vi "Setup UI.vi"(8 "error in (no error)":errorcluster, 10 "Set UI to input? (F)":bool, 11 "PC Reader.lvclass":refnum<class "Photon Counter Reader.lvclass">) -> (0 "error out":errorcluster, 3 "PC Reader out":refnum<class "Photon Counter Reader.lvclass">)   [LabVIEW 2017, in "Photon Counter Reader.lvclass"]
doc: "Setup UI (re)constructs an object -- populates its member data -- from a front panel the user can see. The VI should be as simple as possible so that a UI loop can poll it continuously for updates. \n\nThe VI is designed to be used as a subPanel within another VI. Wire true to \"Set UI to input\" only on the first call, just after inserting this VI into a subPanel, to populate its controls with the class's current values.\n\nSetup UI is distinct from the class constructor. Class constructors are not polymorphic, yet configure dialogs need to configure objects without knowing their type -- and polymorphism is the necessary solution. Thus, Setup UI is a polymorphic class constructor. This continously polled \"Setup UI\" concept is a kludge: a better idea would be an XControl, but those require a steeper learning curve."
uses:
  Photon Counter Reader.lvclass
  Photon Counter Reader.lvclass/Photon Counter Reader.ctl
panel:
  in  "clear template":bool
  in  "Which channels?":u16(ring)=2 items=["A", "B", "A and B", "A, B average"]
  in  "template: Ch A scan":bool
  in  "template: Ch A/B split":bool
  in  "template: continuous scan":bool
  in  "Gate B Ref":enum16{"t=0", "t=T/4", "t=T/2", "t=3T/4"}(ring)
  in  "Gate A Ref":enum16{"t=0", "t=T/4", "t=T/2", "t=3T/4"}(ring)
  out "Gate B Delay Actual":dbl[unit]
  out "Gate A Delay Actual":dbl[unit]
  in  "start vs mid. of gate":bool caption="Delays measured to"
  in  "Gate B %":dbl
  in  "Gate A %":dbl
  in  "time vs percent":bool caption="Width in"
  out "Gate B Mode":enum16{"CW", "Fixed", "Scan"}(ring)
  out "Gate A Mode":enum16{"CW", "Fixed", "Scan"}(ring)
  in  "Gate B Width":dbl[unit]
  in  "Gate B Delay":dbl[unit]
  in  "Gate A Delay":dbl[unit]
  in  "Gate A Width":dbl[unit]
  in  "Ext. Trigger?":bool
  in  "Ext. Trig. Freq.":dbl[unit]=42076.2
  in  "Count Time":dbl[unit]=1.0 format="%#_4g"
  in  "Send first pt to PC":bool
  in  "indAw?":bool
  in  "indAd?":bool
  in  "indBw?":bool
  in  "indBd?":bool
  # "Photon Counter Setup"
  # "Track ind.var.?\n(assumes in ns)"
  # "(PEM = 42.0762 kHz)"
  # "(If tracking, these times represent \nthe values for the first pt.)"
  # "PURE VIRTUAL\nMETHOD CALLED!"
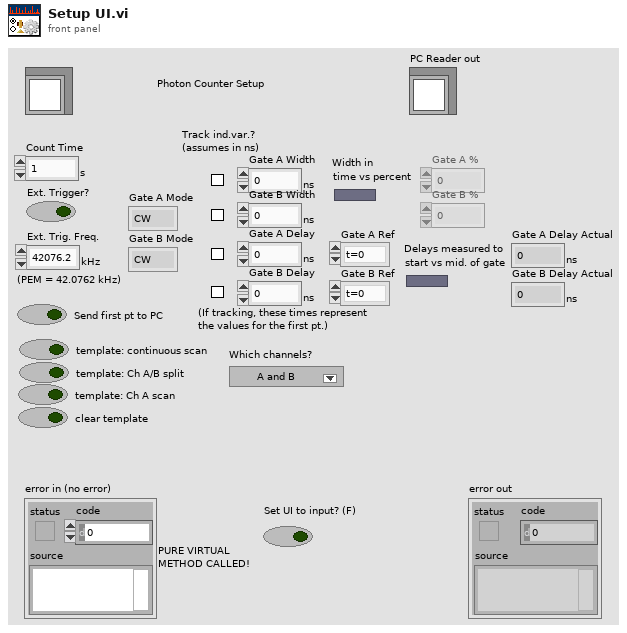
[diagram p1: front panel]
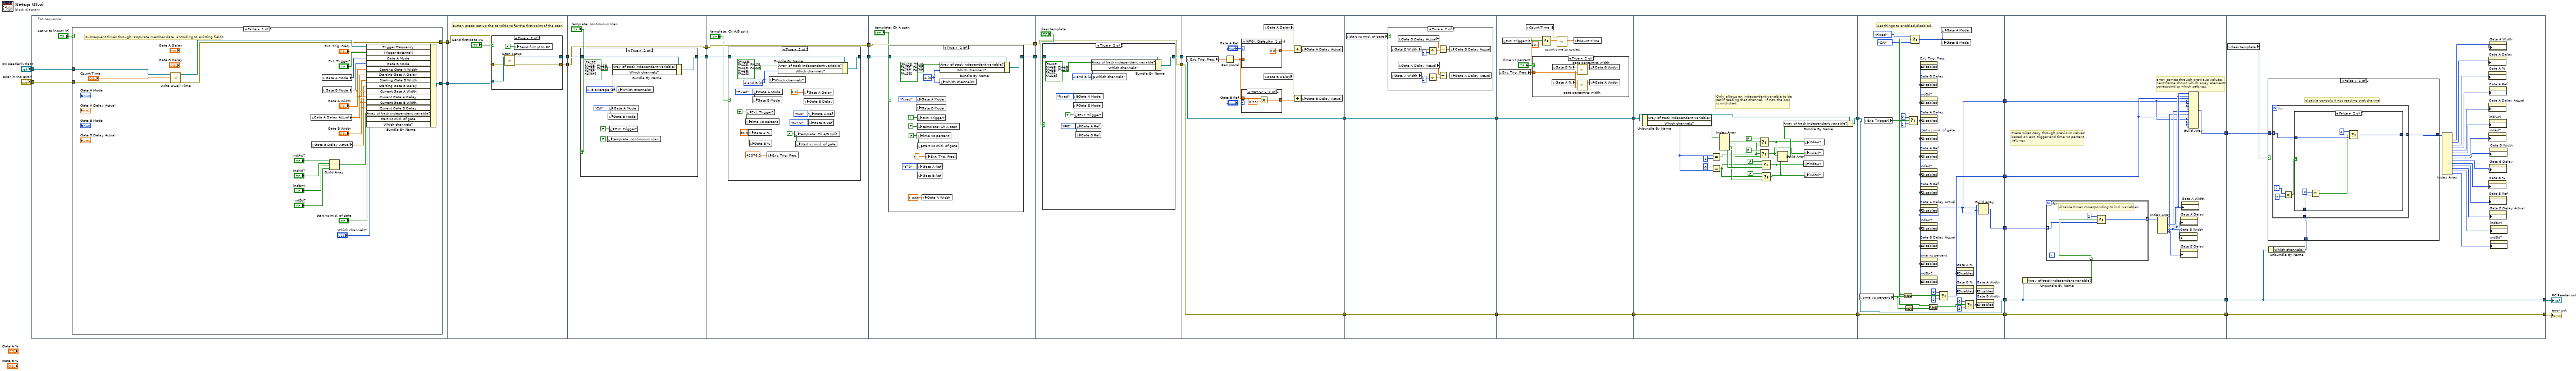
[diagram p0: block diagram]
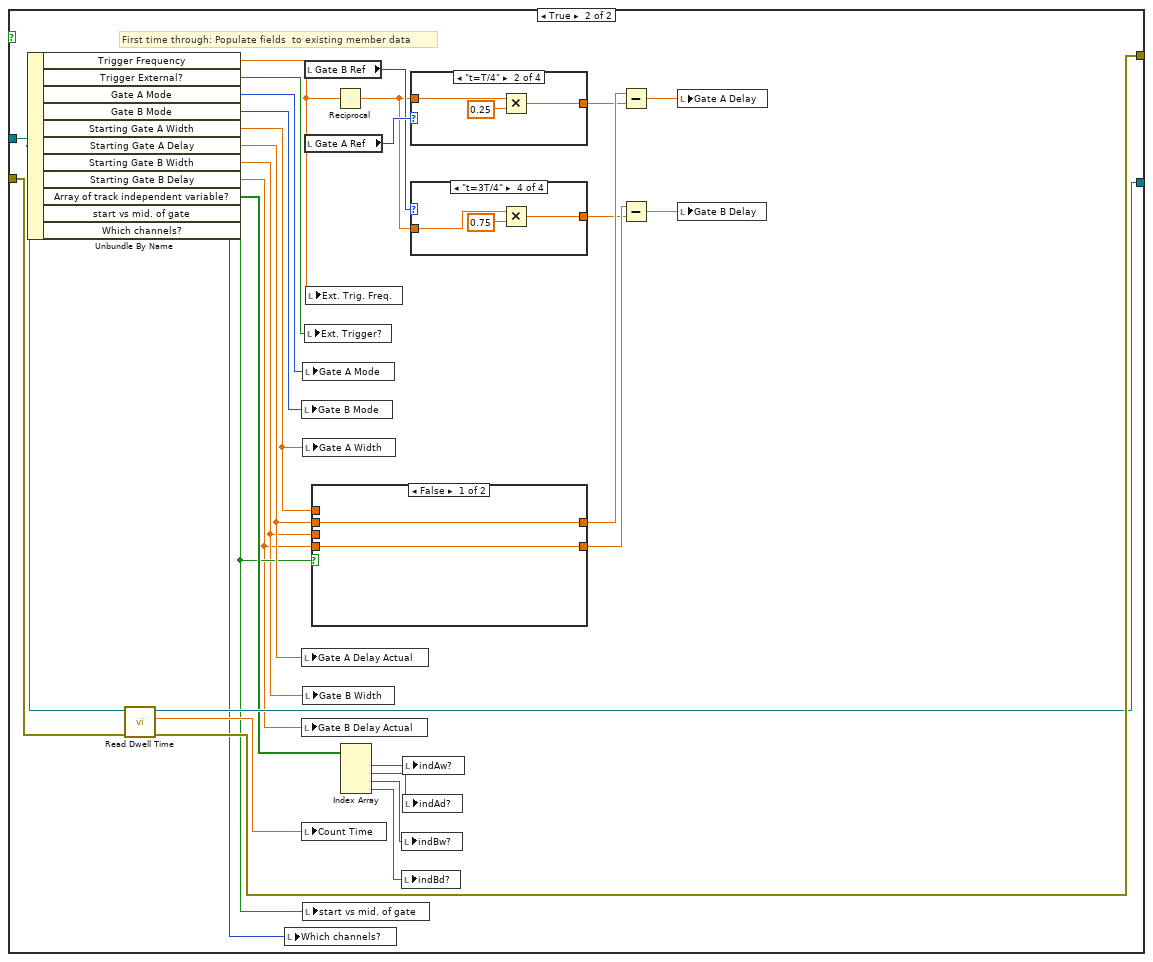
[diagram p2: hidden frame]
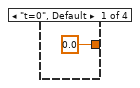
[diagram p3: hidden frame]
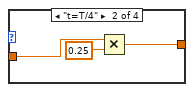
[diagram p4: hidden frame]
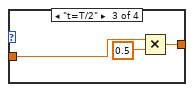
[diagram p5: hidden frame]
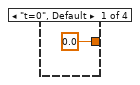
[diagram p6: hidden frame]
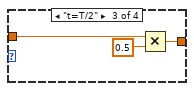
[diagram p7: hidden frame]
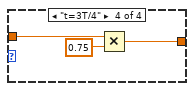
[diagram p8: hidden frame]
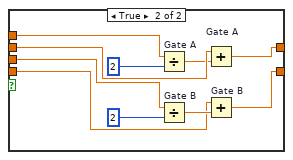
[diagram p9: hidden frame]
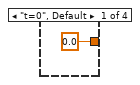
[diagram p15: hidden frame]
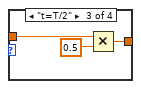
[diagram p16: hidden frame]
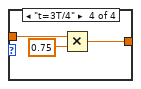
[diagram p17: hidden frame]
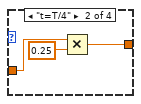
[diagram p18: hidden frame]
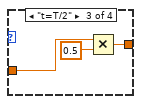
[diagram p19: hidden frame]
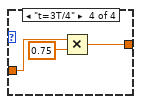
[diagram p20: hidden frame]
diagram:
  n1 = flat-sequence {
    tunnel: "error in (no error)" -> [w34]
    tunnel: [w37] -> w26
    tunnel: [w33] -> w25
    tunnel: "PC Reader.lvclass" -> [w35]
    tunnel: w26 -> [w124]
    tunnel: w25 -> [w123]
    tunnel: [w122] -> w24
    tunnel: [w120] -> w23
    tunnel: w24 -> [w132]
    tunnel: w23 -> [w134]
    tunnel: [w133] -> w22
    tunnel: [w132] -> w21
    tunnel: w22 -> [w145]
    tunnel: [w144] -> w20
    tunnel: w21 -> [w146]
    tunnel: [w146] -> w19
    tunnel: w20 -> [w163]
    tunnel: [w162] -> w4
    tunnel: w19 -> [w164]
    tunnel: [w164] -> w2
    tunnel: w4 -> [w178]
    tunnel: [w179] -> w3
    tunnel: w2 -> [w177]
    tunnel: [w177] -> w1
    tunnel: [w200] -> w29
    tunnel: [w199] -> w28
    tunnel: w3 -> [w199]
    tunnel: w1 -> [w200]
    tunnel: w29 -> [w223]
    tunnel: [w223] -> w31
    tunnel: w28 -> [w222]
    tunnel: [w222] -> w30
    tunnel: w31 -> [w244]
    tunnel: [w244] -> w18
    tunnel: w30 -> [w243]
    tunnel: [w243] -> w16
    tunnel: w18 -> [w276]
    tunnel: [w276] -> w17
    tunnel: w16 -> [w261]
    tunnel: [w260] -> w15
    tunnel: w17 -> [w286]
    tunnel: w15 -> [w285]
    tunnel: [w286] -> w12
    tunnel: [w285] -> w11
    tunnel: [w284] -> w10
    tunnel: [w282] -> w9
    tunnel: [w281] -> w8
    tunnel: w12 -> [w308]
    tunnel: w11 -> [w306]
    tunnel: w10 -> [w304]
    tunnel: w9 -> [w299]
    tunnel: w8 -> [w298]
    tunnel: [w308] -> w7
    tunnel: [w306] -> w6
    tunnel: [w297] -> w5
    tunnel: [w331] -> w13
    tunnel: [w332] -> w14
    tunnel: w7 -> [w332]
    tunnel: w6 -> [w331]
    tunnel: w5 -> [w329]
    frame #0 {
      n2 = case shown="False" "Set UI to input? (F)" {
        tunnel: [w50 w78] -> w37
        tunnel: w35 -> [w51 w79]
        tunnel: [w47 w80] -> w33
        tunnel: w34 -> [w46 w81]
        frame False {
          # "Subsequent times through: Populate member data  according to existing fields"
          n3 = call-dynamic "Write Dwell Time.vi"("error in (no error)"=w46, "Dwell Time"="Count Time", "Reader.lvclass in"=w51) -> ("error out"=w47:errorcluster, "Reader.lvclass out"=w49:refnum<class "Photon Counter Reader.lvclass">)  [unwired: 7 out]
          n4 = local read "Gate A Delay Actual"() -> (w43:dbl[unit])
          n5 = local read "Gate B Delay Actual"() -> (w41:dbl[unit])
          n6 = local read "Gate A Mode"() -> (w52:enum16{"CW", "Fixed", "Scan"})
          n7 = local read "Gate B Mode"() -> (w45:enum16{"CW", "Fixed", "Scan"})
          n8 = Build Array("indAw?", "indAd?", "indBw?", "indBd?") -> (w40:bool[])
          n9 = Bundle By Name(cluster=w49, "Trigger Frequency"="Ext. Trig. Freq.", "Trigger External?"="Ext. Trigger?", "Gate A Mode"=w52, "Gate B Mode"=w45, "Starting Gate A Width"="Gate A Width", "Starting Gate A Delay"=w43, "Starting Gate B Width"="Gate B Width", "Starting Gate B Delay"=w41, "Current Gate A Width"="Gate A Width", "Current Gate A Delay"=w43, "Current Gate B Width"="Gate B Width", "Current Gate B Delay"=w41, "Array of track independent variable?"=w40, "start vs mid. of gate"="start vs mid. of gate", "Which channels?"="Which channels?") -> (w50:refnum<class "Photon Counter Reader.lvclass">)
        }
        frame True {
          # "First time through: Populate fields  to existing member data"
          n10 = Unbundle By Name(w79) -> ("Trigger Frequency"=w74:dbl[unit], "Trigger External?"=w83:bool, "Gate A Mode"=w82:u16, "Gate B Mode"=w68:u16, "Starting Gate A Width"=w66:dbl[unit], "Starting Gate A Delay"=w67:dbl[unit], "Starting Gate B Width"=w63:dbl[unit], "Starting Gate B Delay"=w62:dbl[unit], "Array of track independent variable?"=w65:bool[], "start vs mid. of gate"=w64:bool, "Which channels?"=w59:u16)
          n11 = call-dynamic "Read Dwell Time.vi"("error in (no error)"=w81, "Reader.lvclass in"=w79) -> ("error out"=w80:errorcluster, "Dwell Time"=w77:dbl[unit], "Reader.lvclass out"=w78:refnum<class "Photon Counter Reader.lvclass">)  [unwired: 7 out]
          n12 = local write "Which channels?"(w59) -> ()
          n13 = local write "Gate B Mode"(w68) -> ()
          n14 = local write "Gate A Delay Actual"(w67) -> ()
          n15 = local write "Gate B Delay Actual"(w62) -> ()
          n16 = local write "Count Time"(w77) -> ()
          n17 = local write "Gate A Mode"(w82) -> ()
          n18 = local write "Gate A Width"(w66) -> ()
          n19 = local write "Gate B Width"(w63) -> ()
          n20 = local write "start vs mid. of gate"(w64) -> ()
          n21 = local read "Gate B Ref"() -> (w75:enum16{"t=0", "t=T/4", "t=T/2", "t=3T/4"})
          n22 = local read "Gate A Ref"() -> (w76:enum16{"t=0", "t=T/4", "t=T/2", "t=3T/4"})
          n23 = local write "Ext. Trigger?"(w83) -> ()
          n24 = local write "Ext. Trig. Freq."(w74) -> ()
          n25 = case shown="False" w64 {
            tunnel: [w109 w113] -> w72
            tunnel: w67 -> [w109 w117]
            tunnel: [w108 w112] -> w69
            tunnel: w66 -> [_ w114]
            tunnel: w63 -> [_ w111]
            tunnel: w62 -> [w108 w110]
            frame False {
            }
            frame True {
              n26 = Divide "Gate A"(x=w114, y=2) -> (x/y=w116:dbl[unit])
              n27 = Divide "Gate B"(x=w111, y=2) -> (x/y=w115:dbl[unit])
              n28 = Add "Gate A"(x=w117, y=w116) -> (x+y=w113:dbl[unit])
              n29 = Add "Gate B"(x=w110, y=w115) -> (x+y=w112:dbl[unit])
            }
          }
          n30 = Reciprocal(x=w74) -> (1/x=w73:dbl[unit])
          n31 = Index Array(array=w65) -> (element #1=w84:bool, element #2=w85:bool, element #3=w86:bool, element #4=w87:bool)  [unwired: 4 in]
          n32 = local write "indBw?"(w86) -> ()
          n33 = local write "indBd?"(w87) -> ()
          n34 = local write "indAw?"(w84) -> ()
          n35 = local write "indAd?"(w85) -> ()
          n36 = case shown="\"t=T/4\"" w76 {
            tunnel: [dbl[unit] 0.0 ("x/y") w99 w102 w105] -> w71
            tunnel: w73 -> [_ w100 w103 w106]
            frame "t=0", Default {
            }
            frame "t=T/4" {
              n37 = Multiply(x=w100, y=0.25) -> (x*y=w99:dbl[unit])
            }
            frame "t=T/2" {
              n38 = Multiply(x=w103, y=0.5) -> (x*y=w102:dbl[unit])
            }
            frame "t=3T/4" {
              n39 = Multiply(x=w106, y=0.75) -> (x*y=w105:dbl[unit])
            }
          }
          n40 = case shown="\"t=3T/4\"" w75 {
            tunnel: [dbl[unit] 0.0 ("x/y") w89 w92 w95] -> w60
            tunnel: w73 -> [_ w90 w93 w96]
            frame "t=0", Default {
            }
            frame "t=T/4" {
              n41 = Multiply(x=w90, y=0.25) -> (x*y=w89:dbl[unit])
            }
            frame "t=T/2" {
              n42 = Multiply(x=w93, y=0.5) -> (x*y=w92:dbl[unit])
            }
            frame "t=3T/4" {
              n43 = Multiply(x=w96, y=0.75) -> (x*y=w95:dbl[unit])
            }
          }
          n44 = Subtract(x=w72, y=w71) -> (x-y=w70:dbl[unit])
          n45 = Subtract(x=w69, y=w60) -> (x-y=w61:dbl[unit])
          n46 = local write "Gate A Delay"(w70) -> ()
          n47 = local write "Gate B Delay"(w61) -> ()
        }
      }
    }
    frame #1 {
      # "Button press: set up the conditions for the first point of the scan"
      n48 = case shown="True" "Send first pt to PC" {
        tunnel: [w126 w127] -> w120
        tunnel: [w125 w128] -> w122
        tunnel: w124 -> [w126 w130]
        tunnel: w123 -> [w125 w129]
        frame False {
        }
        frame True {
          n49 = call-dynamic "Scan Setup.vi"("error in (no error)"=w129, "PC Reader in"=w130) -> ("error out"=w128:errorcluster, "PC Reader out"=w127:refnum<class "Photon Counter Reader.lvclass">)  [unwired: 8 out]
          n50 = local write "Send first pt to PC"(FALSE ("Send conds for first point to PG")) -> ()
        }
      }
    }
    frame #2 {
      n51 = case shown="True" "template: continuous scan" {
        tunnel: w134 -> [w136 w142]
        tunnel: [w136 w140] -> w133
        frame False {
        }
        frame True {
          w137 = u16 3 items=["A", "B", "A and B", "A, B average"] ("Which channels?")
          w143 = enum16{"CW", "Fixed", "Scan"}."CW" ("Gate A Mode")
          n52 = local write "template: continuous scan"(FALSE ("template: continuous scan")) -> ()
          n53 = local write "Gate B Mode"(w143) -> ()
          n54 = local write "Gate A Mode"(w143) -> ()
          n55 = local write "Ext. Trigger?"(FALSE ("Ext. Trigger?")) -> ()
          n56 = Bundle By Name(cluster=w142, "Array of track independent variable?"=bool[] [FALSE, FALSE, FALSE, FALSE, FALSE, FALSE, FALSE], "Which channels?"=w137) -> (w140:refnum<class "Photon Counter Reader.lvclass">)
          n57 = local write "Which channels?"(w137) -> ()
        }
      }
    }
    frame #3 {
      n58 = case shown="True" "template: Ch A/B split" {
        tunnel: w145 -> [w148 w160]
        tunnel: [w148 w159] -> w144
        frame False {
        }
        frame True {
          w149 = u16 2 items=["A", "B", "A and B", "A, B average"] ("Which channels?")
          w151 = FALSE ("template: Ch A/B split")
          w155 = dbl[unit] 0.0 ("Gate A Delay")
          w156 = 50.0 ("Gate A %")
          w157 = TRUE ("Ext. Trigger?")
          w158 = enum16{"CW", "Fixed", "Scan"}."Fixed" ("Gate A Mode")
          n59 = local write "time vs percent"(w157) -> ()
          n60 = local write "Ext. Trigger?"(w157) -> ()
          n61 = local write "Gate A %"(w156) -> ()
          n62 = local write "Gate B %"(w156) -> ()
          n63 = local write "Gate B Mode"(w158) -> ()
          n64 = local write "Gate A Mode"(w158) -> ()
          n65 = local write "Ext. Trig. Freq."(dbl[unit] 42076.2 ("Ext. Trig. Freq.")) -> ()
          n66 = local write "Which channels?"(w149) -> ()
          n67 = Bundle By Name(cluster=w160, "Array of track independent variable?"=bool[] [FALSE, FALSE, FALSE, FALSE, FALSE, FALSE, FALSE], "Which channels?"=w149) -> (w159:refnum<class "Photon Counter Reader.lvclass">)
          n68 = local write "template: Ch A/B split"(w151) -> ()
          n69 = local write "start vs mid. of gate"(w151) -> ()
          n70 = local write "Gate A Delay"(w155) -> ()
          n71 = local write "Gate B Delay"(w155) -> ()
          n72 = local write "Gate B Ref"(enum16{"t=0", "t=T/4", "t=T/2", "t=3T/4"}."t=T/2" ("Gate B Ref")) -> ()
          n73 = local write "Gate A Ref"(enum16{"t=0", "t=T/4", "t=T/2", "t=3T/4"}."t=0" ("Gate A Ref")) -> ()
        }
      }
    }
    frame #4 {
      n74 = case shown="True" "template: Ch A scan" {
        tunnel: w163 -> [w165 w176]
        tunnel: [w165 w175] -> w162
        frame False {
        }
        frame True {
          w166 = u16 0 items=["A", "B", "A and B", "A, B average"] ("Which channels?")
          w170 = enum16{"t=0", "t=T/4", "t=T/2", "t=3T/4"}."t=0" ("Gate A Ref")
          w169 = FALSE ("time vs percent")
          w174 = enum16{"CW", "Fixed", "Scan"}."Fixed" ("Gate A Mode")
          n75 = local write "Gate A Mode"(w174) -> ()
          n76 = local write "Gate B Mode"(w174) -> ()
          n77 = local write "time vs percent"(w169) -> ()
          n78 = local write "Ext. Trigger?"(TRUE ("Ext. Trigger?")) -> ()
          n79 = local write "template: Ch A scan"(FALSE ("template: Ch A sweep")) -> ()
          n80 = local write "Gate A Ref"(w170) -> ()
          n81 = local write "Gate B Ref"(w170) -> ()
          n82 = local write "start vs mid. of gate"(w169) -> ()
          n83 = local write "Gate A Width"(dbl[unit] 1.0000000000000002e-06 ("Gate A Width")) -> ()
          n84 = local write "Ext. Trig. Freq."(dbl[unit] 1000.0 ("Ext. Trig. Freq.")) -> ()
          n85 = local write "Which channels?"(w166) -> ()
          n86 = Bundle By Name(cluster=w176, "Array of track independent variable?"=bool[] [FALSE, TRUE, FALSE, FALSE, FALSE, FALSE, FALSE], "Which channels?"=w166) -> (w175:refnum<class "Photon Counter Reader.lvclass">)
        }
      }
    }
    frame #5 {
      n87 = case shown="True" "clear template" {
        tunnel: [w181 w187] -> w179
        tunnel: w178 -> [w181 w188]
        frame False {
        }
        frame True {
          w182 = enum16{"t=0", "t=T/4", "t=T/2", "t=3T/4"}."t=0" ("Gate A Ref")
          w183 = enum16{"CW", "Fixed", "Scan"}."Fixed" ("Gate A Mode")
          w185 = u16 2 items=["A", "B", "A and B", "A, B average"] ("Which channels?")
          n88 = local write "Gate A Mode"(w183) -> ()
          n89 = local write "Gate B Mode"(w183) -> ()
          n90 = local write "Ext. Trigger?"(TRUE ("Ext. Trigger?")) -> ()
          n91 = local write "Gate A Ref"(w182) -> ()
          n92 = local write "Gate B Ref"(w182) -> ()
          n93 = local write "Which channels?"(w185) -> ()
          n94 = Bundle By Name(cluster=w188, "Array of track independent variable?"=bool[] [FALSE, FALSE, FALSE, FALSE, FALSE, FALSE, FALSE], "Which channels?"=w185) -> (w187:refnum<class "Photon Counter Reader.lvclass">)
        }
      }
    }
    frame #6 {
      n95 = local read "Ext. Trig. Freq."() -> (w196:dbl[unit])
      n96 = Reciprocal(x=w196) -> (1/x=w195:dbl[unit])
      n97 = case shown="\"t=0\", Default" "Gate A Ref" {
        tunnel: w195 -> [_ w213 w216 w219]
        tunnel: [dbl[unit] 0.0 ("x/y") w212 w215 w218] -> w193
        frame "t=0", Default {
        }
        frame "t=T/4" {
          n98 = Multiply(x=w213, y=0.25) -> (x*y=w212:dbl[unit])
        }
        frame "t=T/2" {
          n99 = Multiply(x=w216, y=0.5) -> (x*y=w215:dbl[unit])
        }
        frame "t=3T/4" {
          n100 = Multiply(x=w219, y=0.75) -> (x*y=w218:dbl[unit])
        }
      }
      n101 = case shown="\"t=T/4\"" "Gate B Ref" {
        tunnel: w195 -> [_ w203 w206 w209]
        tunnel: [dbl[unit] 0.0 ("x/y") w202 w205 w208] -> w190
        frame "t=0", Default {
        }
        frame "t=T/4" {
          n102 = Multiply(x=w203, y=0.25) -> (x*y=w202:dbl[unit])
        }
        frame "t=T/2" {
          n103 = Multiply(x=w206, y=0.5) -> (x*y=w205:dbl[unit])
        }
        frame "t=3T/4" {
          n104 = Multiply(x=w209, y=0.75) -> (x*y=w208:dbl[unit])
        }
      }
      n105 = local read "Gate A Delay"() -> (w194:dbl[unit])
      n106 = local read "Gate B Delay"() -> (w191:dbl[unit])
      n107 = Add(x=w194, y=w193) -> (x+y=w192:dbl[unit])
      n108 = Add(x=w191, y=w190) -> (x+y=w189:dbl[unit])
      n109 = local write "Gate A Delay Actual"(w192) -> ()
      n110 = local write "Gate B Delay Actual"(w189) -> ()
    }
    frame #7 {
      n111 = local read "start vs mid. of gate"() -> (w221:bool)
      n112 = case shown="True" w221 {
        frame False {
          n113 = local read "Gate B Delay Actual"() -> (w224:dbl[unit])
          n114 = local read "Gate A Delay Actual"() -> (w225:dbl[unit])
          n115 = local write "Gate B Delay Actual"(w224) -> ()
          n116 = local write "Gate A Delay Actual"(w225) -> ()
        }
        frame True {
          n117 = local read "Gate B Width"() -> (w228:dbl[unit])
          n118 = local read "Gate A Width"() -> (w232:dbl[unit])
          n119 = local read "Gate B Delay Actual"() -> (w229:dbl[unit])
          n120 = local read "Gate A Delay Actual"() -> (w233:dbl[unit])
          n121 = Divide(x=w228, y=2) -> (x/y=w230:dbl[unit])
          n122 = Divide(x=w232, y=2) -> (x/y=w231:dbl[unit])
          n123 = Subtract(x=w229, y=w230) -> (x-y=w226:dbl[unit])
          n124 = Subtract(x=w233, y=w231) -> (x-y=w227:dbl[unit])
          n125 = local write "Gate B Delay Actual"(w226) -> ()
          n126 = local write "Gate A Delay Actual"(w227) -> ()
        }
      }
    }
    frame #8 {
      n127 = local read "Ext. Trig. Freq."() -> (w239:dbl[unit])
      n128 = local read "Ext. Trigger?"() -> (w240:bool)
      n129 = local read "Count Time"() -> (w241:dbl[unit])
      n130 = case shown="True" "time vs percent" {
        tunnel: w239 -> [w249 w252]
        frame False {
          n131 = local read "Gate A Width"() -> (w248:dbl[unit])
          n132 = local read "Gate B Width"() -> (w247:dbl[unit])
          n133 = call "gate width to percent.vi"("Trigger Freq"=w249, "Gate width"=w248) -> ("Gate %"=w246:dbl)  [unwired: 1 out]
          n134 = call "gate width to percent.vi"("Trigger Freq"=w249, "Gate width"=w247) -> ("Gate %"=w245:dbl)  [unwired: 1 out]
          n135 = local write "Gate A %"(w246) -> ()
          n136 = local write "Gate B %"(w245) -> ()
        }
        frame True {
          n137 = local read "Gate A %"() -> (w251:dbl)
          n138 = local read "Gate B %"() -> (w250:dbl)
          n139 = call "gate percent to width.vi"("Trigger Freq"=w252, "Gate %"=w250) -> ("Gate width"=w254:dbl[unit])  [unwired: 1 out]
          n140 = call "gate percent to width.vi"("Trigger Freq"=w252, "Gate %"=w251) -> ("Gate width"=w253:dbl[unit])  [unwired: 1 out]
          n141 = local write "Gate B Width"(w254) -> ()
          n142 = local write "Gate A Width"(w253) -> ()
        }
      }
      n143 = Select(t=w239, s=w240, f=dbl[unit] 10000000.0 ("Trigger Freq")) -> (s? t:f=w237:dbl[unit])
      n144 = call "count time to cycles.vi"("Trigger Freq"=w237, "Count Time Set"=w241) -> ("Count Time Current"=w236:dbl[unit])  [unwired: 1 in, 4 out]
      n145 = local write "Count Time"(w236) -> ()
    }
    frame #9 {
      # "Only allows an independent variable to be \nset if reading that channel.  If not, the box\nis unclicked."
      n146 = Unbundle By Name(w261) -> ("Array of track independent variable?"=w275:bool[], "Which channels?"=w270:u16)
      n147 = Equal?(x=w270, y=u16 1) -> (x = y?=w262:bool)
      n148 = Equal?(x=u16 0, y=w270) -> (x = y?=w267:bool)
      n149 = Index Array(array=w275) -> (element #1=w274:bool, element #2=w273:bool, element #3=w272:bool, element #4=w271:bool)  [unwired: 4 in]
      n150 = Select(t=FALSE, s=w262, f=w274) -> (s? t:f=w256:bool)
      n151 = Select(t=FALSE, s=w262, f=w273) -> (s? t:f=w255:bool)
      n152 = Select(t=FALSE, s=w267, f=w272) -> (s? t:f=w257:bool)
      n153 = Select(t=FALSE, s=w267, f=w271) -> (s? t:f=w258:bool)
      n154 = Build Array(w256, w255, w257, w258) -> (w259:bool[])
      n155 = Bundle By Name(cluster=w261, "Array of track independent variable?"=w259) -> (w260:refnum<class "Photon Counter Reader.lvclass">)
      n156 = local write "indBw?"(w257) -> ()
      n157 = local write "indAw?"(w256) -> ()
      n158 = local write "indAd?"(w255) -> ()
      n159 = local write "indBd?"(w258) -> ()
    }
    frame #10 {
      # "Set things to enabled/disabled."
      n160 = local read "time vs percent"() -> (w287:bool)
      n161 = local read "Ext. Trigger?"() -> (w280:bool)
      n162 = And(x=w280, y=w287) -> (x .and. y?=w292:bool)
      n163 = Not(x=w287) -> (.not. x?=w288:bool)
      n164 = Select(t=0, s=w280, f=2) -> (s? t:f=w281:i32)
      n165 = Select(t=enum16{"CW", "Fixed", "Scan"}."Fixed" ("Gate A Mode"), s=w280, f=enum16{"CW", "Fixed", "Scan"}."CW" ("Gate A Mode")) -> (s? t:f=w277:enum16{"CW", "Fixed", "Scan"})
      n166 = property on="Ext. Trig. Freq." class="DigNum (strict)"("Disabled"=w281) -> ()  [unwired: 2 in, 2 out]
      n167 = property on="Gate B Delay" class="DigNum (strict)"("Disabled"=w281) -> ()  [unwired: 2 in, 2 out]
      n168 = property on="indBd?" class="Bool (strict)"("Disabled"=w281) -> ()  [unwired: 2 in, 2 out]
      n169 = property on="Gate A Delay" class="DigNum (strict)"("Disabled"=w281) -> ()  [unwired: 2 in, 2 out]
      n170 = property on="start vs mid. of gate" class="Bool (strict)"("Disabled"=w281) -> ()  [unwired: 2 in, 2 out]
      n171 = property on="Gate A Ref" class="Enum (strict)"("Disabled"=w281) -> ()  [unwired: 2 in, 2 out]
      n172 = property on="indAd?" class="Bool (strict)"("Disabled"=w281) -> ()  [unwired: 2 in, 2 out]
      n173 = property on="Gate B Ref" class="Enum (strict)"("Disabled"=w281) -> ()  [unwired: 2 in, 2 out]
      n174 = property on="Gate A Delay Actual" class="DigNum (strict)"("Disabled"=w281) -> ()  [unwired: 2 in, 2 out]
      n175 = property on="indAw?" class="Bool (strict)"("Disabled"=w281) -> ()  [unwired: 2 in, 2 out]
      n176 = property on="Gate B Delay Actual" class="DigNum (strict)"("Disabled"=w281) -> ()  [unwired: 2 in, 2 out]
      n177 = property on="time vs percent" class="Bool (strict)"("Disabled"=w281) -> ()  [unwired: 2 in, 2 out]
      n178 = property on="indBw?" class="Bool (strict)"("Disabled"=w281) -> ()  [unwired: 2 in, 2 out]
      n179 = And(x=w280, y=w288) -> (x .and. y?=w289:bool)
      n180 = Select(t=0, s=w292, f=2) -> (s? t:f=w282:i32)
      n181 = local write "Gate B Mode"(w277) -> ()
      n182 = local write "Gate A Mode"(w277) -> ()
      n183 = property on="Gate A %" class="DigNum (strict)"("Disabled"=w282) -> ()  [unwired: 2 in, 2 out]
      n184 = property on="Gate B %" class="DigNum (strict)"("Disabled"=w282) -> ()  [unwired: 2 in, 2 out]
      n185 = Select(t=0, s=w289, f=2) -> (s? t:f=w283:i32)
      n186 = property on="Gate A Width" class="DigNum (strict)"("Disabled"=w283) -> ()  [unwired: 2 in, 2 out]
      n187 = property on="Gate B Width" class="DigNum (strict)"("Disabled"=w283) -> ()  [unwired: 2 in, 2 out]
      n188 = Build Array(w283, w281, w283, w281) -> (w284:i32[])
    }
    frame #11 {
      # "these wires carry through previous values\nbased on ext. trigger and time vs percent\nsettings."
      # "array carries through previous values.\nnext frame shows which array elements\ncorrespond to which settings."
      n189 = Unbundle By Name(w306) -> ("Array of track independent variable?"=w305:bool[])
      n190 = for {
        tunnel: [w309] -> w307 mode=indexing
        tunnel: w305 -> [w312] mode=indexing
        tunnel: w304 -> [w311] mode=indexing
        # "disable times corresponding to ind. variables"
        n191 = Select(t=2, s=w312, f=w311) -> (s? t:f=w309:i32)
      }
      n192 = Index Array(array=w307) -> (element #1=w303:i32, element #2=w302:i32, element #3=w301:i32, element #4=w300:i32)  [unwired: 4 in]
      n193 = property on="Gate B Width" class="DigNum (strict)"("DisabledEnum"=w301) -> ()  [unwired: 2 in, 2 out]
      n194 = property on="Gate A Delay" class="DigNum (strict)"("DisabledEnum"=w302) -> ()  [unwired: 2 in, 2 out]
      n195 = property on="Gate B Delay" class="DigNum (strict)"("DisabledEnum"=w300) -> ()  [unwired: 2 in, 2 out]
      n196 = property on="Gate A Width" class="DigNum (strict)"("DisabledEnum"=w303) -> ()  [unwired: 2 in, 2 out]
      n197 = Build Array(w303, w302, w299, w298, w298, w298, w298, w301, w300, w299, w298, w298, w298, w298) -> (w297:i32[])
    }
    frame #12 {
      n198 = local read "clear template"() -> (w313:bool)
      n199 = Unbundle By Name(w331) -> ("Which channels?"=w330:u16)
      n200 = case shown="False" w313 {
        tunnel: w330 -> [w335 _]
        tunnel: w329 -> [w334 w363]
        tunnel: [w333 w354] -> w328
        frame False {
          # "disable controls if not reading that channel"
          n201 = for {
            tunnel: w335 -> [w338]
            tunnel: w334 -> [w339] mode=indexing
            tunnel: [w337] -> w333 mode=indexing
            i -> [w336]
            n202 = Less?(x=w336, y=7) -> (x < y?=w340:bool)
            n203 = case shown="False" w340 {
              tunnel: w339 -> [w347 w353]
              tunnel: w338 -> [w346 w352]
              tunnel: [w342 w348] -> w337
              frame True {
                n204 = Equal?(x=u16 1, y=w346) -> (x = y?=w344:bool)
                n205 = Select(t=2, s=w344, f=w347) -> (s? t:f=w342:i32)
              }
              frame False {
                n206 = Equal?(x=u16 0, y=w352) -> (x = y?=w350:bool)
                n207 = Select(t=2, s=w350, f=w353) -> (s? t:f=w348:i32)
              }
            }
          }
        }
        frame True {
          # "If open template is selected, this enables all controls exept for\ngate width and %.  The enabling/disabling of these controls is \nchecked earlier and by the time vs. percent swtich and is carried\nthrough here."
          n208 = Initialize Array(0, 14 ("dimension size")) -> (w364:i32[])
          n209 = Index Array(array=w363, index #1=0 ("index"), index #2=2 ("index"), index #3=7 ("index"), index #4=9 ("index")) -> (element #1=w355:i32, element #2=w356:i32, element #3=w357:i32, element #4=w358:i32)
          n210 = local write "clear template"(FALSE ("open template")) -> ()
          n211 = Replace Array Subset(array=w364, new element #1=w355, index #1=0 ("index"), new element #2=w356, index #2=2 ("index"), new element #3=w357, index #3=7 ("index"), new element #4=w358, index #4=9 ("index")) -> (w354:i32[])
        }
      }
      n212 = Index Array(array=w328) -> (element #1=w327:i32, element #2=w326:i32, element #3=w325:i32, element #4=w324:i32, element #5=w323:i32, element #6=w322:i32, element #7=w321:i32, element #8=w320:i32, element #9=w319:i32, element #10=w318:i32, element #11=w317:i32, element #12=w316:i32, element #13=w315:i32, element #14=w314:i32)  [unwired: 14 in]
      n213 = property on="Gate A Delay" class="DigNum (strict)"("DisabledEnum"=w326) -> ()  [unwired: 2 in, 2 out]
      n214 = property on="Gate A %" class="DigNum (strict)"("DisabledEnum"=w325) -> ()  [unwired: 2 in, 2 out]
      n215 = property on="Gate A Delay Actual" class="DigNum (strict)"("DisabledEnum"=w323) -> ()  [unwired: 2 in, 2 out]
      n216 = property on="indAd?" class="Bool (strict)"("DisabledEnum"=w321) -> ()  [unwired: 2 in, 2 out]
      n217 = property on="Gate B %" class="DigNum (strict)"("DisabledEnum"=w318) -> ()  [unwired: 2 in, 2 out]
      n218 = property on="Gate A Ref" class="Enum (strict)"("DisabledEnum"=w324) -> ()  [unwired: 2 in, 2 out]
      n219 = property on="indAw?" class="Bool (strict)"("DisabledEnum"=w322) -> ()  [unwired: 2 in, 2 out]
      n220 = property on="Gate B Ref" class="Enum (strict)"("DisabledEnum"=w317) -> ()  [unwired: 2 in, 2 out]
      n221 = property on="Gate A Width" class="DigNum (strict)"("DisabledEnum"=w327) -> ()  [unwired: 2 in, 2 out]
      n222 = property on="Gate B Delay" class="DigNum (strict)"("DisabledEnum"=w319) -> ()  [unwired: 2 in, 2 out]
      n223 = property on="Gate B Delay Actual" class="DigNum (strict)"("DisabledEnum"=w316) -> ()  [unwired: 2 in, 2 out]
      n224 = property on="Gate B Width" class="DigNum (strict)"("DisabledEnum"=w320) -> ()  [unwired: 2 in, 2 out]
      n225 = property on="indBw?" class="Bool (strict)"("DisabledEnum"=w315) -> ()  [unwired: 2 in, 2 out]
      n226 = property on="indBd?" class="Bool (strict)"("DisabledEnum"=w314) -> ()  [unwired: 2 in, 2 out]
    }
  }
  "error out" <- w14
  "PC Reader out" <- w13
